vi "Write Front Panel ref.vi"(8 "error in (no error)":errorcluster, 10 "Front Panel ref":refnum<vi>, 11 "Measure Object in":refnum<class "Template Module.lvclass">) -> (0 "error out":errorcluster, 3 "Measure Object out":refnum<class "Template Module.lvclass">)   [LabVIEW 2018, in "Template Module.lvclass"]
uses:
  Template Module.lvclass
  Template Module.lvclass/Template Module.ctl
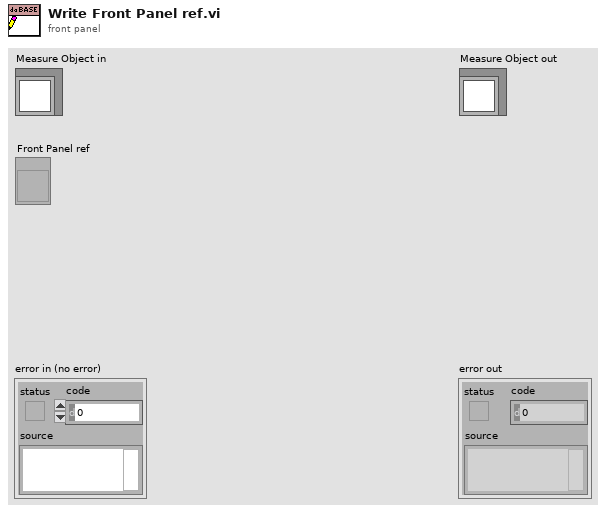
[diagram p1: front panel]
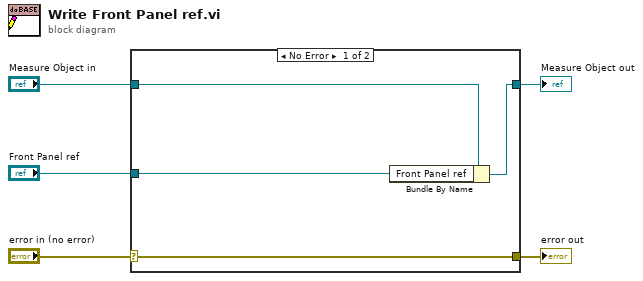
[diagram p0: block diagram]
diagram:
  n1 = case shown="No Error" "error in (no error)" {
    selector: "error in (no error)" -> [w9 w10]
    tunnel: [w9 w10] -> w4
    tunnel: [w7 w11] -> w2
    tunnel: "Measure Object in" -> [w8 w11]
    tunnel: "Front Panel ref" -> [w6 _]
    frame No Error {
      n2 = Bundle By Name(cluster=w8, "Front Panel ref"=w6) -> (w7:refnum<class "Template Module.lvclass">)
    }
    frame Error {
    }
  }
  "error out" <- w4
  "Measure Object out" <- w2
